vi "FPGA IO mapping.vi"() -> ()   [LabVIEW 2014]
uses:
  <vilib>/Platform/TimedLoop/XDataNode/timing_clust.ctl
  <vilib>/Platform/TimedLoop/XDataNode/nitl_modes.ctl
  <vilib>/Platform/TimedLoop/XDataNode/wakeup.ctl
  <vilib>/rvi/Emulation/niFpgaSctlEmulationGetInTimedLoop.vi
  <vilib>/rvi/Emulation/niFpgaEmulationReportErrorSimple.vi
  <vilib>/rvi/Emulation/niFpgaGetClockAttributes.vi
  <vilib>/rvi/Emulation/niFpgaCriticalErrorInLSC.vi
  <vilib>/rvi/Emulation/niFpgaProcessEmulError.vi
  <vilib>/Platform/TimedLoop/XDataNode/XDataNode.xnode
  <vilib>/Platform/TimedLoop/XDataNode/XDNodeRunTimeDep.lvlib
  <vilib>/NI Veristand/FPGA/NI_VS FPGA Support.lvlib
  <userlib>/_NI VeriStand FPGA Support/NI VeriStand FPGA Clock Support/NI_VS FPGA Clock Support.lvlib
panel:
  in  "_PWM Pulses 4-7":u64[](array[numeric])=[0, 0, 0, 0]
  in  "_PWM Pulses 0-3":u64[](array[numeric])=[0, 0, 0, 0]
  in  "Generate IRQ":bool
  in  "Use External Timing":bool
  in  "Write to  RTSI":bool
  in  "Loop Rate (usec)":u32
  in  "Start":bool
  # "PWM"
  # "Configuration"
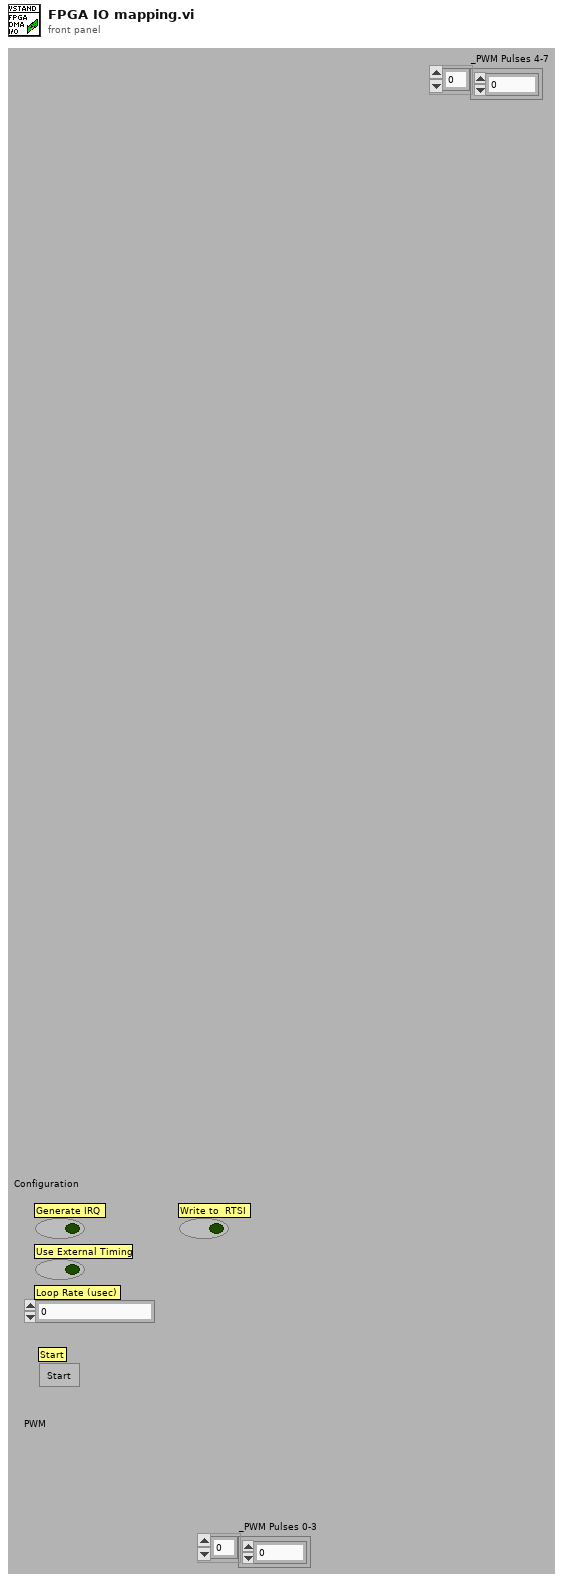
[diagram p1: front panel]
types:
  T1 = typedef "XDNodeRunTimeDep.lvlib/timing_clust.ctl" = cluster{"Expected End [f-1]":u64, "Actual End [f-1]":u64, "Finished Late? [f-1]":bool, "Expected End [i-1]":u64, "Actual End [i-1]":u64, "Finished Late? [i-1]":bool, "Expected Start [i]":u64, "Actual Start [i]":u64, "Expected Start [f]":u64, "Actual Start [f]":u64, "Source Name":string, "Structure Name":string, "Period":i64, "Deadline":i64, "Offset":i64, "Start":i64, "Priority":i32, "Timeout":i32, "Mode":T2, "Wakeup Reason":T3, "Error":errorcluster, "Source Type":string, "Secondary Source Type":string, "Global End Time":u64, "Global Start Time":u64, "Frame Duration":u64, "Iteration Duration":u64, "Assigned CPU":i32, "I/O Scan Engine Mode":u32}
  T2 = typedef "XDNodeRunTimeDep.lvlib/nitl_modes.ctl" = enum32{"No Change", "Process missed periods, maintain original phase", "Discard missed periods, maintain original phase", "Process missed periods, ignore original phase", "Discard missed periods, ignore original phase"}
  T3 = typedef "XDNodeRunTimeDep.lvlib/wakeup.ctl" = enum32{"Normal", "Aborted", "Asynchronous wakeup", "Timing source error", "Timed loop error", "Timeout"}
  T4 = cluster{"AO0":refnum<k21>, "AO1":refnum<k21>, "AO2":refnum<k21>, "AO3":refnum<k21>}
  T5 = cluster{"9215 AI0":refnum<k21>, "9215 AI1":refnum<k21>, "9215 AI2":refnum<k21>, "9215 AI3":refnum<k21>}
  T6 = cluster{"DO0":refnum<k21>, "DO1":refnum<k21>, "DO2":refnum<k21>, "DO3":refnum<k21>}
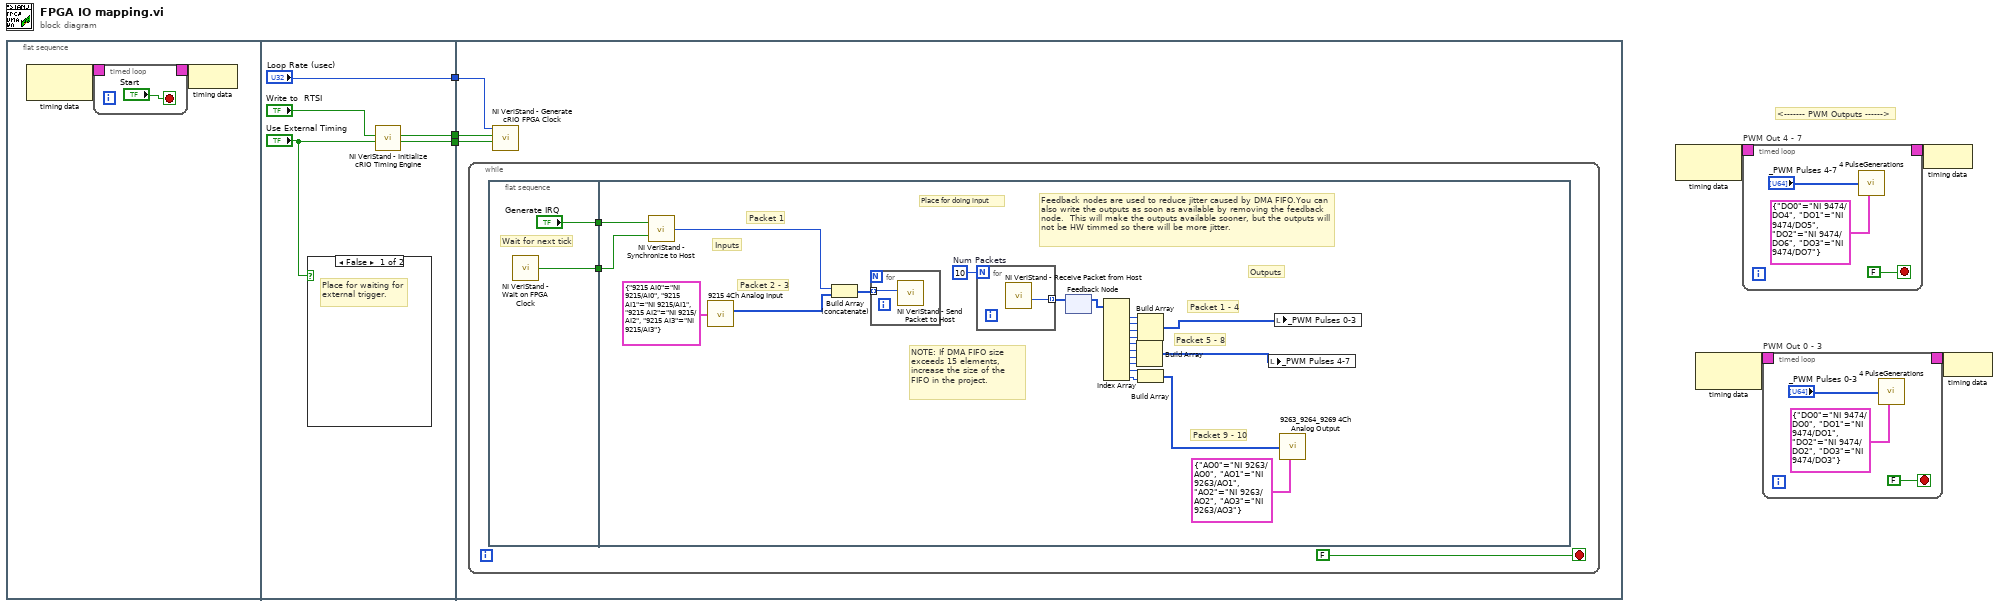
[diagram p0: block diagram]
diagram:
  # "<------- PWM Outputs ------>"
  n1 = flat-sequence {
    tunnel: [w16] -> w7
    tunnel: ["Loop Rate (usec)"] -> w6
    tunnel: [w15] -> w3
    tunnel: w7 -> [w22]
    tunnel: w6 -> [w21]
    tunnel: w3 -> [w20]
    frame #0 {
      n2 = node-c288() -> (w9:T1)  [unwired: 1 out]
      n3 = timed-loop {
        timing: w9 -> [_]
        timing-out: [_] -> w8
        stop <- "Start" stop-if-true
      }
      n4 = node-c288(w8) -> ()
    }
    frame #1 {
      n5 = case shown="False" "Use External Timing" {
        frame False {
          # "Place for waiting for external trigger."
        }
        frame True {
          # "Do not wait on trigger when externally timed."
        }
      }
      n6 = call <userlib>:"NI VeriStand - Initialize cRIO Timing Engine.vi"("Use External Timing In"="Use External Timing", "Write to  RTSI In"="Write to  RTSI") -> ("Use External Timing Out"=w16:bool, "Write to  RTSI Out"=w15:bool)  [unwired: 8 in]
    }
    frame #2 {
      n7 = while {
        stop <- FALSE stop-if-true
        n8 = flat-sequence {
          tunnel: ["Generate IRQ"] -> w24
          tunnel: [w26] -> w23
          tunnel: w24 -> [w50]
          tunnel: w23 -> [w49]
          frame #0 {
            # "Wait for next tick"
            n9 = call <userlib>:"NI VeriStand - Wait on FPGA Clock.vi"() -> ("Clock Ticked"=w26:bool)
          }
          frame #1 {
            w48 = 10  # Num Packets
            # "Packet 5 - 8"
            # "Packet 1"
            # "Packet 2 - 3"
            # "Inputs"
            # "Outputs"
            # "Packet 9 - 10"
            # "Packet 1 - 4"
            # "NOTE: If DMA FIFO size exceeds 15 elements, increase the size of the FIFO in the project."
            # "Feedback nodes are used to reduce jitter caused by DMA FIFO.You can also write the outputs as soon as available by removing the feedback node.  This will make the outputs available sooner, but the outputs will not be HW timmed so there will be more jitter."
            # "Place for doing input"
            n10 = call <userlib>:"NI VeriStand - Synchronize to Host.vi"("Clock Ticked"=w49, "Generate IRQ"=w50) -> ("Is Late?"=w36:u64)
            n11 = call <userlib>:"9215 4Ch Analog Input.vi"("9215 I/O"=T5 {"9215 AI0"="NI 9215/AI0", "9215 AI1"="NI 9215/AI1", "9215 AI2"="NI 9215/AI2", "9215 AI3"="NI 9215/AI3"}) -> ("Packets"=w35:u64[])
            n12 = Build Array (concatenate)(w36, w35) -> (w43:u64[])
            n13 = for {
              tunnel: w43 -> [w51] mode=indexing
              n14 = call <vilib>:"NI VeriStand - Send Packet to Host.vi"("Element"=w51) -> ()  [unwired: 2 in, 9 out]
            }
            n15 = for {
              N: w48 -> [_]
              tunnel: [w52] -> w40 mode=indexing
              n16 = call <vilib>:"NI VeriStand - Receive Packet from Host.vi"() -> ("Element"=w52:u64)  [unwired: 2 in, 9 out]
            }
            n17 = feedback-in #1(w40) -> ()
            n18 = feedback #1() -> (w41:u64[])  [unwired: 1 in]
            n19 = Index Array(array=w41) -> (element #1=w47:u64, element #2=w46:u64, element #3=w45:u64, element #4=w44:u64, element #5=w32:u64, element #6=w31:u64, element #7=w30:u64, element #8=w29:u64, element #9=w34:u64, element #10=w33:u64)  [unwired: 10 in]
            n20 = Build Array(w32, w31, w30, w29) -> (w28:u64[])
            n21 = Build Array(w47, w46, w45, w44) -> (w42:u64[])
            n22 = Build Array(w34, w33) -> (w38:u64[])
            n23 = local write "_PWM Pulses 4-7"(w28) -> ()
            n24 = local write "_PWM Pulses 0-3"(w42) -> ()
            n25 = call <userlib>:"9263_9264_9269 4Ch Analog Output.vi"("Packets"=w38, "9263/4/9 I/O"=T4 {"AO0"="NI 9263/AO0", "AO1"="NI 9263/AO1", "AO2"="NI 9263/AO2", "AO3"="NI 9263/AO3"}) -> ()  [unwired: 8 in]
          }
        }
      }
      n26 = call <userlib>:"NI VeriStand - Generate cRIO FPGA Clock.vi"("Use External Timing"=w22, "Write to  RTSI"=w20, "Loop Rate (usec)"=w21) -> ()  [unwired: 9 in]
    }
  }
  n27 = node-c288() -> (w2:T1)  [unwired: 1 out]
  n28 = node-c288() -> (w5:T1)  [unwired: 1 out]
  n29 = timed-loop "PWM Out 4 - 7" {
    timing: w2 -> [_]
    timing-out: [_] -> w1
    stop <- FALSE stop-if-true
    n30 = call <userlib>:"4 PulseGenerations.vi"("PulseGen Packets"="_PWM Pulses 4-7", "4 PulseGen Chs"=T6 {"DO0"="NI 9474/DO4", "DO1"="NI 9474/DO5", "DO2"="NI 9474/DO6", "DO3"="NI 9474/DO7"}) -> ()  [unwired: 8 in]
  }
  n31 = timed-loop "PWM Out 0 - 3" {
    timing: w5 -> [_]
    timing-out: [_] -> w4
    stop <- FALSE stop-if-true
    n32 = call <userlib>:"4 PulseGenerations.vi"("PulseGen Packets"="_PWM Pulses 0-3", "4 PulseGen Chs"=T6 {"DO0"="NI 9474/DO0", "DO1"="NI 9474/DO1", "DO2"="NI 9474/DO2", "DO3"="NI 9474/DO3"}) -> ()  [unwired: 8 in]
  }
  n33 = node-c288(w1) -> ()
  n34 = node-c288(w4) -> ()
